vi "Open Hardware.vi"(8 "error in (no error)":errorcluster, 11 "Instrument.VRM in":refnum<class "Instrument.OxfordVRM.lvclass">) -> (0 "error out":errorcluster, 3 "Instrument.VRM out":refnum<class "Instrument.OxfordVRM.lvclass">)   [LabVIEW 2019, in "Instrument.OxfordVRM.lvclass"]
uses:
  Instrument.OxfordVRM.lvclass
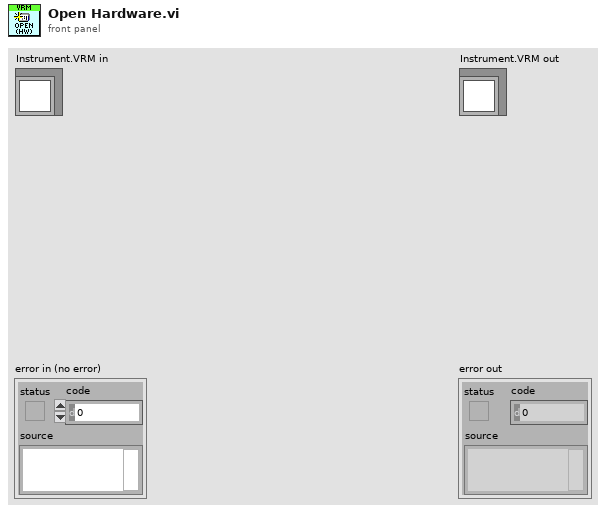
[diagram p1: front panel]
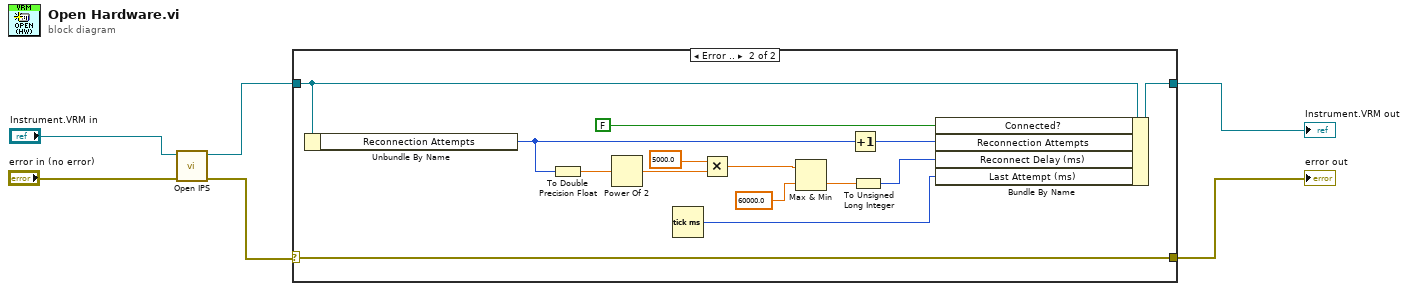
[diagram p0: block diagram]
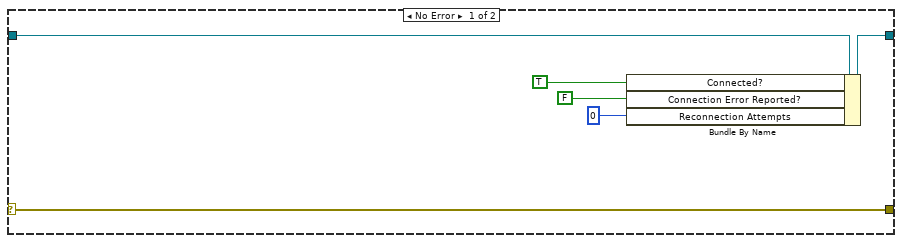
[diagram p2: hidden frame]
diagram:
  n1 = call "Open IPS.vi"("error in (no error)"="error in (no error)", "Instrument.OxfordVRM in"="Instrument.VRM in") -> ("error out"=w3:errorcluster, "Instrument.OxfordVRM out"=w4:refnum<class "Instrument.OxfordVRM.lvclass">)  [unwired: 8 in]
  n2 = case shown="Error .." w3 {
    selector: w3 -> [w12 w26]
    tunnel: [w12 w26] -> w2
    tunnel: w4 -> [w8 w23]
    tunnel: [w7 w24] -> w1
    frame No Error {
      n3 = Bundle By Name(cluster=w8, "Connected?"=TRUE ("Connection.Connected?"), "Connection Error Reported?"=FALSE ("Connection.Connection Error Reported?"), "Reconnection Attempts"=u32 0 ("Connection.Reconnection Attempts")) -> (w7:refnum<class "Instrument.OxfordVRM.lvclass">)
    }
    frame Error {
      n4 = Unbundle By Name(w23) -> ("Reconnection Attempts"=w15:u32)
      n5 = To Double Precision Float(number=w15) -> (double precision float=w19:dbl)
      n6 = Power Of 2(x=w19) -> (2^x=w16:dbl)
      n7 = Tick Count (ms)() -> (millisecond timer value=w17:u32)
      n8 = Multiply(x=5000.0 ("Connection.Reconnection Attempts"), y=w16) -> (x*y=w18:dbl)
      n9 = Max & Min(x=w18, y=60000.0 ("Connection.Reconnection Attempts")) -> (min(x,y)=w22:dbl)  [unwired: 1 out]
      n10 = Increment(x=w15) -> (x+1=w14:u32)
      n11 = To Unsigned Long Integer(number=w22) -> (unsigned 32bit integer=w13:u32)
      n12 = Bundle By Name(cluster=w23, "Connected?"=FALSE ("Connection.Connected?"), "Reconnection Attempts"=w14, "Reconnect Delay (ms)"=w13, "Last Attempt (ms)"=w17) -> (w24:refnum<class "Instrument.OxfordVRM.lvclass">)
    }
  }
  "error out" <- w2
  "Instrument.VRM out" <- w1
